vi "tsc--Color Picker Simulator.vi"() -> ()   [LabVIEW 2021]
uses:
  a3999398-c5a3-4985-9eac-f53f14a1d766.vi
  User32.dll
panel:
  out "Color start":u32(colorbox)
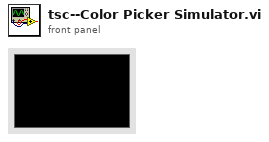
[diagram p1: front panel]
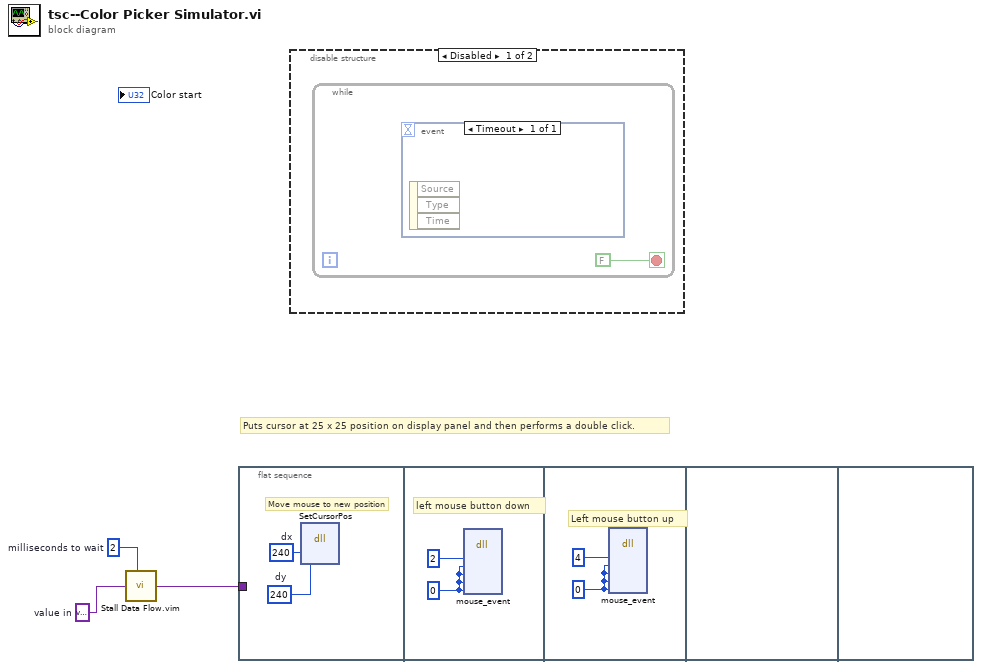
[diagram p0: block diagram]
diagram:
  w3 = variant  # value in
  w2 = u32 2  # milliseconds to wait
  # "Puts cursor at 25 x 25 position on display panel and then performs a double click."
  n1 = call "Stall Data Flow.vim"("value in"=w3, "milliseconds to wait"=w2) -> ("value out"=w1:variant)  [unwired: 1 out]
  n2 = flat-sequence {
    tunnel: w1 -> [_]
    frame #0 {
      w5 = 240  # dy
      w4 = 240  # dx
      # "Move mouse to new position"
      n3 = dll-call lib="User32.dll" fn="SetCursorPos" label="Move mouse to new pos"("dx"=w4, "dy"=w5) -> ()  [unwired: 6 in, 2 out]
    }
    frame #1 {
      w7 = u32 0 ("dy")
      # "left mouse button down"
      n4 = dll-call lib="user32.dll" fn="mouse_event"("dwFlags"=u32 2, "dx"=w7, "dy"=w7, "dwData"=w7, "dwExtraInfo"=w7) -> ()  [unwired: 9 in, 2 out]
    }
    frame #2 {
      w9 = u32 0 ("dy")
      # "Left mouse button up"
      n5 = dll-call lib="user32.dll" fn="mouse_event"("dwFlags"=u32 4, "dx"=w9, "dy"=w9, "dwData"=w9, "dwExtraInfo"=w9) -> ()  [unwired: 9 in, 2 out]
    }
    frame #3 {
    }
    frame #4 {
    }
  }
  n6 = disable-structure shown="Disabled" {
    frame Disabled {
      n7 = while {
        stop <- FALSE stop-if-true
        n8 = event shown="[0] Timeout" {
          selector: _ -> [_]
          dyn-events: _ -> [_]
          timeout: _ -> [_]
          event Timeout {
            n9 = event-data() -> ()  [unwired: 1 in, 3 out]
          }
        }
      }
    }
    frame Enabled {
    }
  }
